vi "MOKE Labview for B115 PMOKE.vi"() -> ()   [LabVIEW 2020]
panel:
  in  "Loop":dbl
  in  "Kepco Curr Step (A)":dbl
  in  "Max Kepco Curr (A)":dbl
  in  "Kepco BOP 36-12M GPIB Addr":string
  in  "Model 475 GPIB Addr":string
  in  "Model 2182 GPIB Addr":string
  out "Averaged Result":cluster{"X":dbl, "Y":dbl}[](graph)
  out "Ongoing Measurement":cluster{"X":dbl, "Y":dbl}[](graph)
  in  "stop":bool
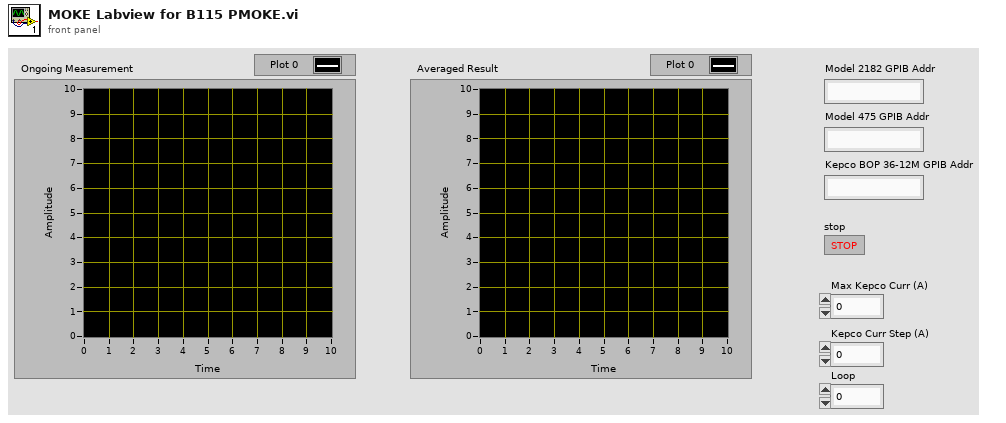
[diagram p1: front panel]
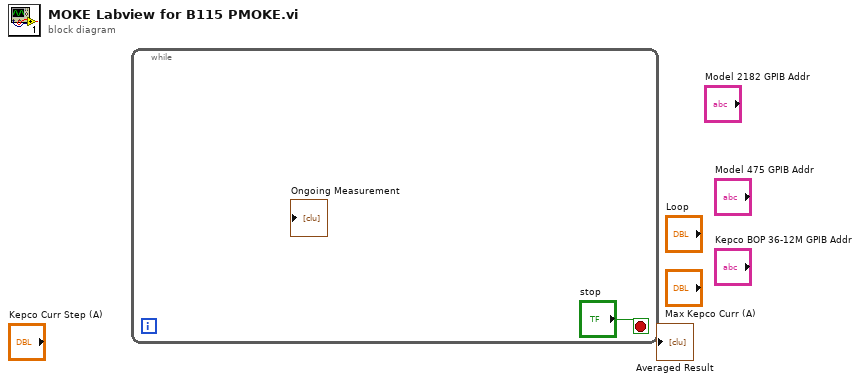
[diagram p0: block diagram]
diagram:
  n1 = while {
    stop <- "stop" stop-if-true
  }
